vi "Initialize DPIDs Cluster.vi"(7 "PID Lookup":variant, 8 "error in":errorcluster, 9 "DPID Lookup":variant, 10 "UUDT Receive ID":u32=513 format="%.0x", 11 "cluster in":refnum<k21>) -> (0 "error out":errorcluster, 1 "DPID Lookup Out":variant, 2 "GMLAN DPID Session":refnum<k21>, 3 "Cluster Out":refnum<k21>)   [LabVIEW 2015, in "Diagnostics Addon Engine.lvlib"]
uses:
  Diagnostics Addon Engine.lvlib
  Shared/CAN Frame.ctl
  Shared/DPID Lookup Cluster.ctl
  Shared/DPID Lookup PID Information.ctl
  Shared/Datatable Lookup Positions.ctl
  Shared/GUID Lookup.vi
  Shared/Diagnostics Addon Shared.lvlib
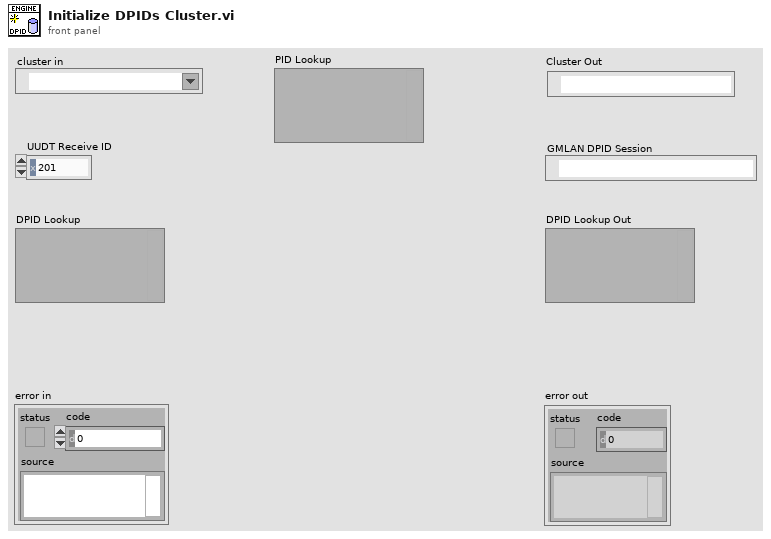
[diagram p1: front panel]
types:
  T1 = typedef "Diagnostics Addon Shared.lvlib/CAN Frame.ctl" = cluster{"Frame name":string, "Identifier":u32, "Payload Length":u32, "Timing Type":u32, "Transmit Time":dbl, "Extended Identifier?":bool, "Comment":string}
  T2 = typedef "Diagnostics Addon Shared.lvlib/DPID Lookup Cluster.ctl" = cluster{"PID Info":T3, "Datatable Lookup":T4, "Conversion":refnum<k21>}
  T3 = typedef "Diagnostics Addon Shared.lvlib/DPID Lookup PID Information.ctl" = cluster{"PID":u16, "Frame Length":u8}
  T4 = typedef "Diagnostics Addon Shared.lvlib/Datatable Lookup Positions.ctl" = cluster{"Offset":i32, "Length":i32}
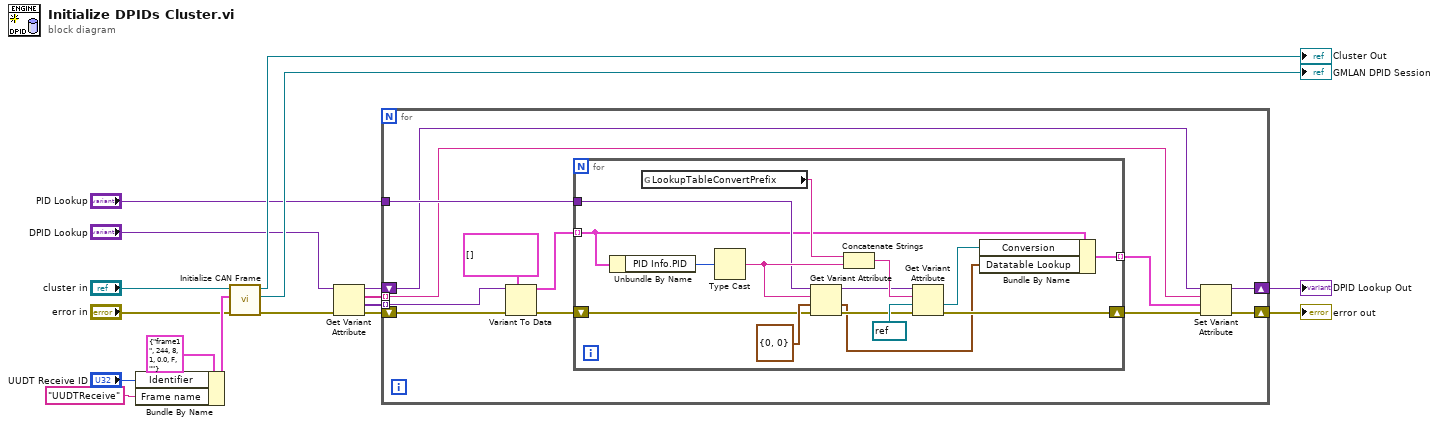
[diagram p0: block diagram]
diagram:
  n1 = Bundle By Name(cluster=T1 {"Frame name"="frame1", "Identifier"=244, "Payload Length"=8, "Timing Type"=1, "Transmit Time"=0.0, "Extended Identifier?"=FALSE, "Comment"=""} ("CAN Frame"), "Identifier"="UUDT Receive ID", "Frame name"="UUDTReceive") -> (w15:T1)
  n2 = call "Initialize CAN Frame.vi"("error in"="error in", "CAN Frame"=w15, "cluster in"="cluster in") -> ("error out"=w2:errorcluster, "frame out"=→"GMLAN DPID Session":refnum<k21>, "cluster out"=→"Cluster Out":refnum<k21>)  [unwired: 6 in]
  n3 = Get Variant Attribute(Variant="DPID Lookup", error in=w2) -> (duplicate Variant=w4:variant, names=w5:string[], values=w8:variant[], error out=w7:errorcluster)  [unwired: 2 in]
  n4 = for {
    tunnel: w8 -> [w28] mode=indexing
    tunnel: "PID Lookup" -> [w24]
    tunnel: w5 -> [w18] mode=indexing
    shift-right: [w19] -> w3
    shift-left: w4 -> [w20]
    shift-right: [w22] -> w1
    shift-left: w7 -> [w29]
    n5 = Variant To Data(error in=w29, type=T2[] [], Variant=w28) -> (data=w26:T2[], error out=w25:errorcluster)
    n6 = for {
      tunnel: w26 -> [w30] mode=indexing
      shift-right: [w35] -> w23
      shift-left: w25 -> [w39]
      tunnel: w24 -> [w37]
      tunnel: [w31] -> w21 mode=indexing
      n7 = Unbundle By Name(w30) -> ("PID Info.PID"=w32:u16)
      n8 = global read "GUID Lookup.vi" "LookupTableConvertPrefix"() -> (w42:string)
      n9 = Type Cast(x=w32) -> (*(type *) &x=w38:string)  [unwired: 1 in]
      n10 = Get Variant Attribute(Variant=w37, name=w38, default value (empty Variant)=T4 {"Offset"=0, "Length"=0} ("cluster"), error in=w39) -> (duplicate Variant=w36:variant, value=w33:T4, error out=w40:errorcluster)  [unwired: 1 out]
      n11 = Concatenate Strings(w42, w38) -> (w43:string)
      n12 = Get Variant Attribute(Variant=w36, name=w43, default value (empty Variant)=refnum<k21> refnum ("DID Conversion"), error in=w40) -> (value=w34:refnum<k21>, error out=w35:errorcluster)  [unwired: 2 out]
      n13 = Bundle By Name(cluster=w30, "Conversion"=w34, "Datatable Lookup"=w33) -> (w31:T2)
    }
    n14 = Set Variant Attribute(Variant=w20, name=w18, value=w21, error in=w23) -> (Variant out=w19:variant, error out=w22:errorcluster)  [unwired: 1 out]
  }
  "error out" <- w1
  "DPID Lookup Out" <- w3
